vi "NewVITemplate.vi"() -> ()   [LabVIEW 2012, in "Body.lvclass"]
uses:
  Body.lvclass
  Bodies.lvclass
panel:
  out "Bodies.lvclass":refnum<class "Bodies.lvclass">
  in  "Bodies.lvclass":refnum<class "Bodies.lvclass">
  out "error out":errorcluster
  in  "error in (no error)":errorcluster
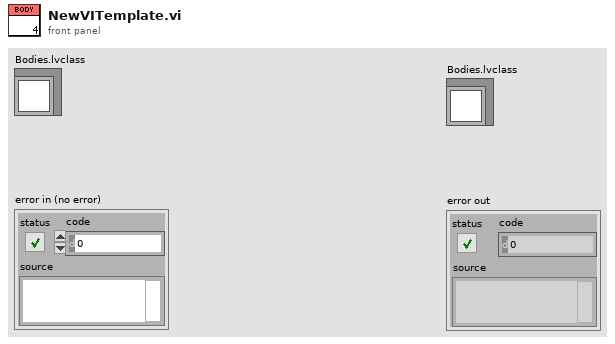
[diagram p1: front panel]
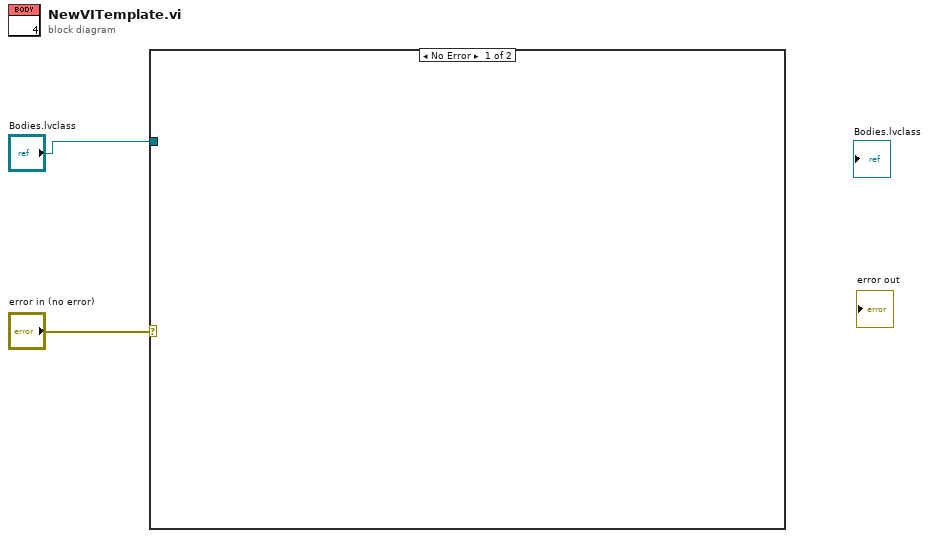
[diagram p0: block diagram]
diagram:
  n1 = case shown="No Error" "error in (no error)" {
    tunnel: "Bodies.lvclass" -> [_ _]
    frame No Error {
    }
    frame Error {
    }
  }
